vi "CC Alarm Object.vi"(8 "error in (no error)":errorcluster, 9 "Alarm":T1, 10 "Source":string, 11 "Alarm Action":T2) -> (0 "error out":errorcluster, 1 "key already included?":bool, 2 "Alarm List":T1[](array[typedef]), 3 "Alarm?":bool)   [LabVIEW 2024]
uses:
  typedefs/CC cluster Alarm Data.ctl
  typedefs/CC enum Alarm Action.ctl
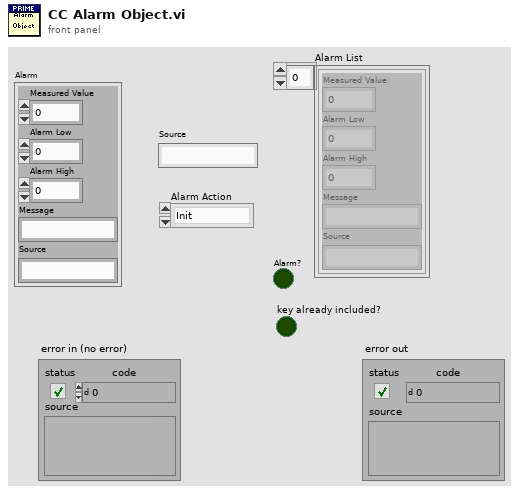
[diagram p1: front panel]
types:
  T1 = typedef "CC cluster Alarm Data.ctl" = cluster{"Measured Value":dbl, "Alarm Low":dbl, "Alarm High":dbl, "Message":string, "Source":string}
  T2 = typedef "CC enum Alarm Action.ctl" = enum16{"Init", "Add Alarm", "Get Alarms", "Clear Alarm", "Clear All Alarms"}
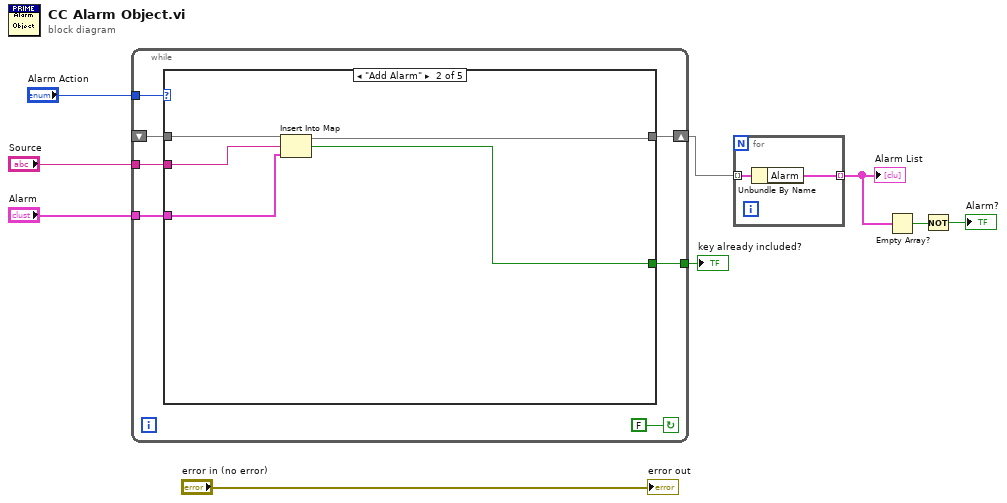
[diagram p0: block diagram]
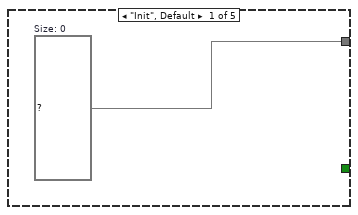
[diagram p2: hidden frame]
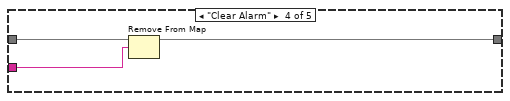
[diagram p4: hidden frame]
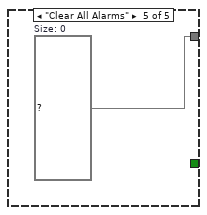
[diagram p5: hidden frame]
diagram:
  n1 = while {
    tunnel: "Alarm Action" -> [w15]
    shift-right: [w14] -> w5
    shift-left: _ -> [w13]
    tunnel: "Source" -> [w12]
    tunnel: "Alarm" -> [w11]
    tunnel: [w10] -> w1
    stop <- FALSE continue-if-true
    n2 = case shown="\"Add Alarm\"" w15 {
      tunnel: [w17 w19 w23 w24 w27] -> w14
      tunnel: w13 -> [_ w22 w23 w26 _]
      tunnel: w12 -> [_ w21 _ w25 _]
      tunnel: w11 -> [_ w20 _ _ _]
      tunnel: [_ w18 _ _ _] -> w10
      frame "Init", Default {
        w17 = map{string, T1} {}  # Size: 0
      }
      frame "Add Alarm" {
        n3 = Insert Into Map(map in=w22, key=w21, value=w20) -> (map out=w19:map{string, T1}, key already included?=w18:bool)  [unwired: 1 out]
      }
      frame "Get Alarms" {
      }
      frame "Clear Alarm" {
        n4 = Remove From Map(10:w25, 11:w26) -> (3:w24:map{string, T1})  [unwired: 2 out]
      }
      frame "Clear All Alarms" {
        w27 = map{string, T1} {}  # Size: 0
      }
    }
  }
  "key already included?" <- w1
  n5 = for {
    tunnel: w5 -> [w29] mode=indexing
    tunnel: [w28] -> w4 mode=indexing
    n6 = Unbundle By Name(w29) -> ("Alarm"=w28:T1)
  }
  "Alarm List" <- w4
  n7 = Empty Array?(array=w4) -> (empty?=w3:bool)
  n8 = Not(x=w3) -> (.not. x?=→"Alarm?":bool)
  "error out" <- "error in (no error)"
